vi "Shutdown.vi"(8 "error in":errorcluster, 11 "nCRD in":refnum<class "nCRD.lvclass">) -> (0 "error out":errorcluster, 3 "nCRD out":refnum<class "nCRD.lvclass">)   [LabVIEW 2014, in "nCRD.lvclass"]
uses:
  nCRD.lvclass
  Session/Raw FPGA/FPGA Session.lvclass
  nCRD.lvclass/nCRD.ctl
  Reusable/CRDS/Main/CRDS.lvclass
  <userlib>/_Session Fwk/Session - Root.lvclass
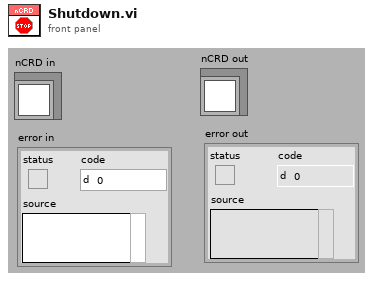
[diagram p1: front panel]
types:
  T1 = typedef "Session - Root.lvclass/Session Handle.ctl" = refnum<data-value>
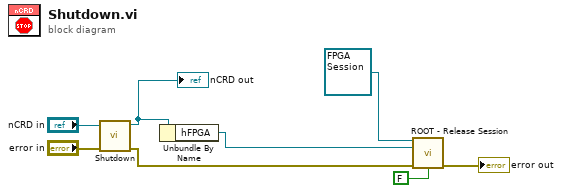
[diagram p0: block diagram]
diagram:
  n1 = call-parent "Shutdown.vi"("error in"="error in", "Instrument in"="nCRD in") -> ("error out"=w1:errorcluster, "Instrument out"=w6:refnum<class "nCRD.lvclass">)  [unwired: 8 in]
  "nCRD out" <- w6
  n2 = Unbundle By Name(w6) -> ("hFPGA"=w5:T1)
  n3 = call <userlib>:"ROOT - Release Session.vi"("OBJ - Session in"=refnum<class "FPGA Session.lvclass"> refnum ("FPGA Session"), "Session Handle in"=w5, "error in (no error)"=w1, "force destroy? (F)"=FALSE) -> ("error out"=→"error out":errorcluster)  [unwired: 9 in, 2 out]
